vi "Test Move Panel.vi"() -> ()   [LabVIEW 2019]
uses:
  Window Mover/Window Mover.lvlib
panel:
  in  "stop":bool
  # "Click and drag to move this panel."
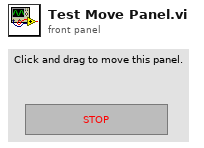
[diagram p1: front panel]
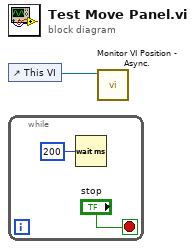
[diagram p0: block diagram]
diagram:
  n1 = control-ref of="This VI"() -> (w1:refnum<vi>)
  n2 = while {
    stop <- "stop" stop-if-true
    n3 = Wait (ms)(milliseconds to wait=u32 200) -> ()  [unwired: 1 out]
  }
  n4 = call "Monitor VI Position - Async..vi"("VI ref."=w1) -> ()  [unwired: 11 in]
